vi "Set IPS Action.vi"(6 "Axis":T1=enum."Z", 8 "error in (no error)":errorcluster, 10 "PSU Act Stat":T2="HOLD" caption="PSU Action Status", 11 "Instrument.OxfordVRM in":refnum<class "Instrument.OxfordVRM.lvclass">) -> (0 "error out":errorcluster, 2 "Response":string, 3 "Instrument.OxfordVRM out":refnum<class "Instrument.OxfordVRM.lvclass">)   [LabVIEW 2019, in "Instrument.OxfordVRM.lvclass"]
uses:
  Instrument.OxfordVRM.lvclass
  <instrlib>/Mercury iXX/Public/Libraries/Magnet/Controls/PSU Actions.ctl
  <userlib>/LevyLab/Instrument Framework/Instrument Types/Cryostat/Typedefs/Magnet Axis--Enum.ctl
  Instrument.OxfordVRM.lvclass/Instrument.OxfordVRM.ctl
  <instrlib>/Mercury iXX/Public/Libraries/Magnet/Open/Open Magnet Device.vi
  <instrlib>/Mercury iXX/Public/Libraries/Magnet/Configuration/Set/PSU Action Status (Set).vi
  <instrlib>/Mercury iXX/Public/Libraries/Magnet/Configuration/Read/PSU Action Status (Read).vi
  <instrlib>/Mercury iXX/Mercury iXX.lvlib
  <instrlib>/Mercury iXX/Public/Libraries/Magnet.lvlib
  <userlib>/LevyLab/Instrument Framework/Instrument Types/Cryostat/Instrument.Cryostat.lvclass
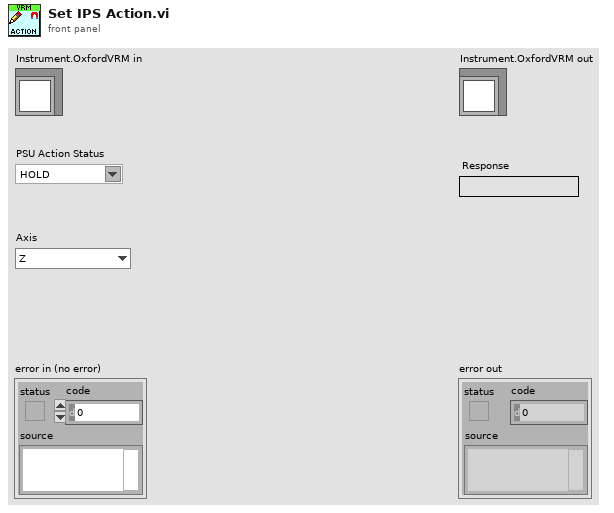
[diagram p1: front panel]
types:
  T1 = typedef "Instrument.Cryostat.lvclass/Magnet Axis--Enum.ctl" = enum16{"X", "Y", "Z"}
  T2 = typedef "Mercury iXX.lvlib/Magnet.lvlib/PSU Actions.ctl" = string
  T3 = typedef "Mercury iXX.lvlib/Mercury Reference.ctl" = cluster{"Comms":refnum<visa-resource-name>, "Device ID":string[], "Comms Layer":T4, "Command":string, "Query reference":T5}
  T4 = typedef "Mercury iXX.lvlib/Comms Transport Layer.ctl" = enum16{"Ethernet TCP/IP", "USB", "ISOBus - RS-232", "GPIB"}
  T5 = typedef "Mercury iXX.lvlib/Query Dynamic Reference.ctl" = refnum<vi>
  T6 = typedef "Mercury iXX.lvlib/Response String.ctl" = string
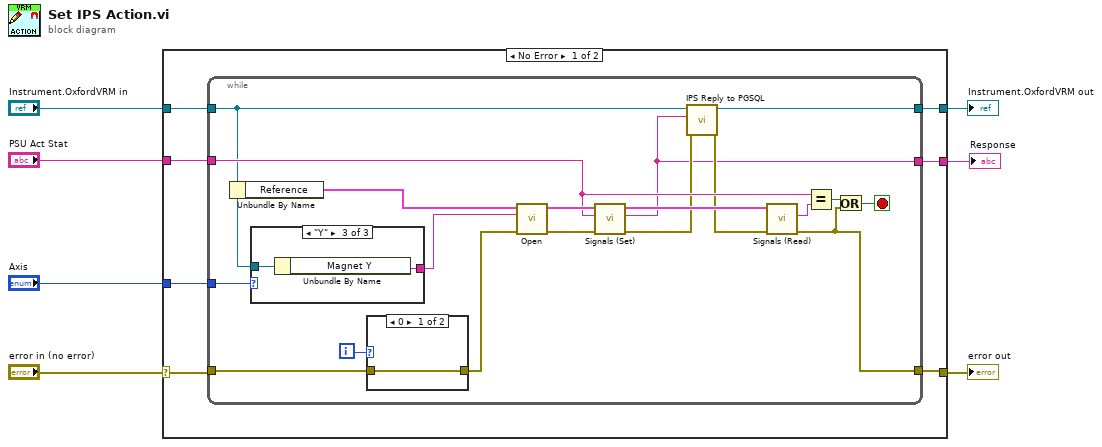
[diagram p0: block diagram]
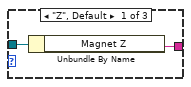
[diagram p2: hidden frame]
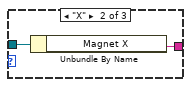
[diagram p3: hidden frame]
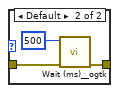
[diagram p4: hidden frame]
diagram:
  n1 = case shown="No Error" "error in (no error)" {
    selector: "error in (no error)" -> [w13 w45]
    tunnel: [w11 w45] -> w6
    tunnel: [w8 w44] -> w4
    tunnel: "Instrument.OxfordVRM in" -> [w14 w44]
    tunnel: [w12 _] -> w3
    tunnel: "PSU Act Stat" -> [w10 _]
    tunnel: "Axis" -> [w9 _]
    frame No Error {
      n2 = while {
        tunnel: w14 -> [w22]
        tunnel: [w15] -> w12
        tunnel: w10 -> [w29]
        tunnel: w9 -> [w20]
        tunnel: [w19] -> w8
        tunnel: w13 -> [w27]
        tunnel: [w16] -> w11
        i -> [w26]
        stop <- w24 stop-if-true
        n3 = Unbundle By Name(w22) -> ("Reference"=w33:T3)
        n4 = case shown="\"Y\"" w20 {
          tunnel: [w35 w37 w39] -> w21
          tunnel: w22 -> [w34 w36 w38]
          frame "Z", Default {
            n5 = Unbundle By Name(w34) -> ("Magnet Z"=w35:string)
          }
          frame "X" {
            n6 = Unbundle By Name(w36) -> ("Magnet X"=w37:string)
          }
          frame "Y" {
            n7 = Unbundle By Name(w38) -> ("Magnet Y"=w39:string)
          }
        }
        n8 = case shown="0" w26 {
          tunnel: w27 -> [w40 w43]
          tunnel: [w40 w42] -> w23
          frame 0 {
          }
          frame Default {
            n9 = call <userlib>:"Wait (ms)__ogtk.vi"("error in (no error)"=w43, "milliseconds to wait"=u32 500) -> ("error out"=w42:errorcluster)  [unwired: 8 in, 1 out]
          }
        }
        n10 = call-poly <instrlib>:"Open.vi"("error in (no error)"=w23, "Device Identifier"=w21, "Mercury Reference In"=w33) -> ("error out"=w31:errorcluster, "Mercury Reference Out"=w32:T3)  [unwired: 7 out]
        n11 = call-poly <instrlib>:"Signals (Set).vi"("error in"=w31, "PSU Act Stat"=w29, "Mercury Reference In"=w32) -> ("error out"=w18:errorcluster, "Response"=w15:T6, "Mercury Reference Out"=w30:T3)  [unwired: 1 in, 5 out]
        n12 = call "IPS Reply to PGSQL.vi"("error in (no error)"=w18, "Response"=w15, "Instrument.VRM in"=w22) -> ("error out"=w17:errorcluster, "Instrument.VRM out"=w19:refnum<class "Instrument.OxfordVRM.lvclass">)  [unwired: 7 in]
        n13 = call-poly <instrlib>:"Signals (Read).vi"("error in"=w17, "Mercury Reference In"=w30) -> ("error out"=w16:errorcluster, "PSU Act Stat"=w28:T2)  [unwired: 1 in, 7 out]
        n14 = Equal?(x=w29, y=w28) -> (x = y?=w25:bool)
        n15 = Or(x=w25, y=w16) -> (x .or. y?=w24:bool)
      }
    }
    frame Error {
    }
  }
  "error out" <- w6
  "Instrument.OxfordVRM out" <- w4
  "Response" <- w3
